vi "TemperatureSensorStart.vi"(0 "Device Info":T1={"Serial Number"=-1, "Channel"=0, "Port"=0}, 1 "Data Interval":i32=-1, 2 "Change Trigger":dbl, 5 "ThermocoupleType":u32(ring)=2 items=["THERMOCOUPLE_TYPE_J"=1, "THERMOCOUPLE_TYPE_K"=2, "THERMOCOUPLE_TYPE_E"=3, "THERMOCOUPLE_TYPE_T"=4], 7 "RTD Type":u32(ring)=2 items=["RTD_TYPE_PT100_3850"=1, "RTD_TYPE_PT1000_3850"=2, "RTD_TYPE_PT100_3920"=3, "RTD_TYPE_PT1000_3920"=4], 9 "RTD Wire Setup":u32(ring)=3 items=["RTD_WIRE_SETUP_2WIRE"=1, "RTD_WIRE_SETUP_3WIRE"=2, "RTD_WIRE_SETUP_4WIRE"=3], 11 "error in (no error)":errorcluster, 12 "Connection":u16(ring) items=["No Preference", "Remote", "Local"], 13 "Timeout (mSec)":i32=5000) -> (4 "Phidget ID":u64, 6 "Serial Number Return":i32, 10 "Attached?":bool, 15 "error out":errorcluster)   [LabVIEW 2012, in "Phidget Temperature Sensor.lvlib"]
doc: "${TemperatureSensor:StartHeader}"
uses:
  <instrlib>/Phidgets/Phidget Temperature Sensor/Phidget Temperature Sensor.lvlib
  <instrlib>/Phidgets/Phidget Common/Phidget Common.lvlib
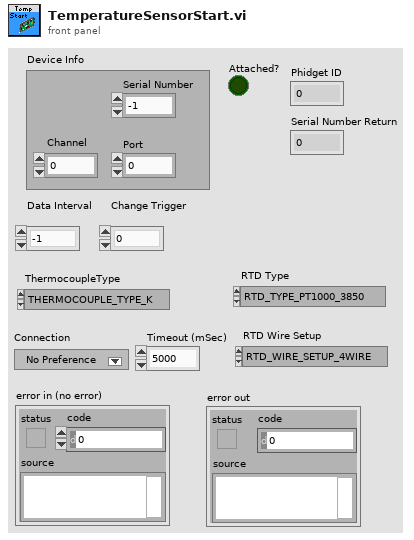
[diagram p1: front panel]
types:
  T1 = cluster{"Serial Number":i32, "Channel":i32, "Port":i32}
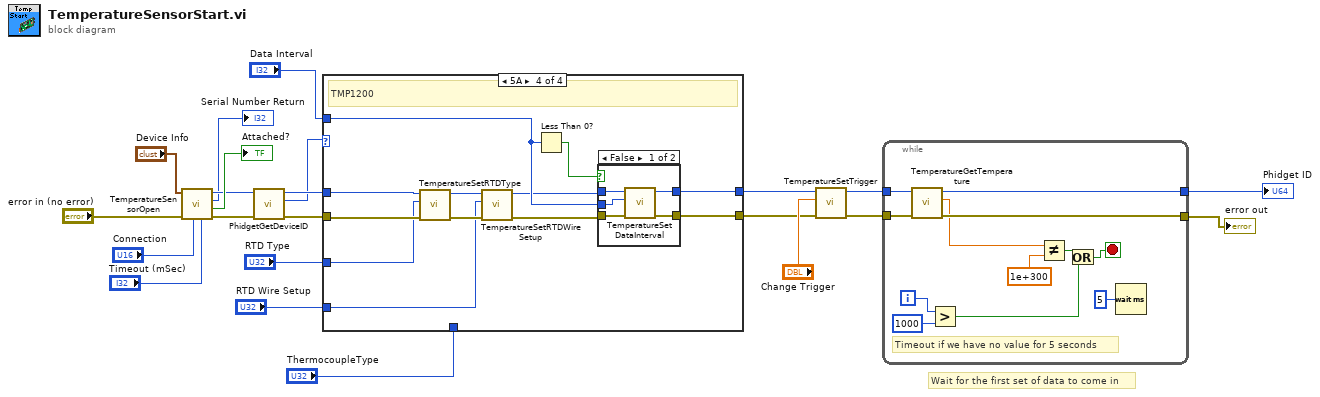
[diagram p0: block diagram]
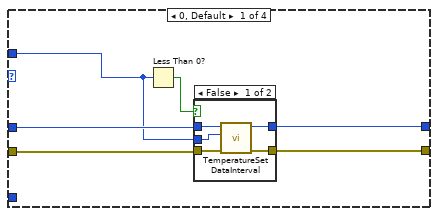
[diagram p2: hidden frame]
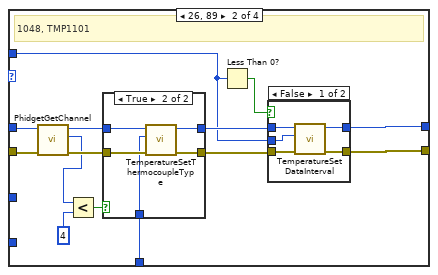
[diagram p4: hidden frame]
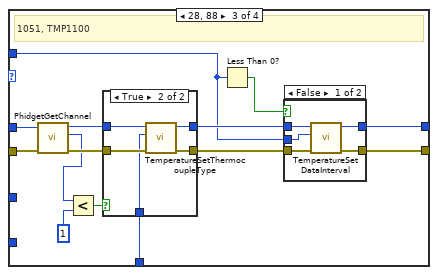
[diagram p7: hidden frame]
diagram:
  # "Wait for the first set of data to come in"
  n1 = call <instrlib>:"TemperatureSensorOpen.vi"("Timeout (mSec)"="Timeout (mSec)", "Connection"="Connection", "error in"="error in (no error)", "Device Info"="Device Info") -> ("error out"=w19:errorcluster, "Attached?"=→"Attached?":bool, "Serial Number Return"=→"Serial Number Return":i32, "Phidget ID"=w18:u64)  [unwired: 4 in]
  n2 = call <instrlib>:"PhidgetGetDeviceID.vi"("error in (no error)"=w19, "Device In"=w18) -> ("error out"=w12:errorcluster, "Devie IDs"=w11:u32, "Device Out"=w13:u64)  [unwired: 6 in]
  n3 = case shown="5A" w11 {
    tunnel: w13 -> [w27 w49 w72 w99]
    tunnel: w12 -> [w26 w48 w71 w96]
    tunnel: [w24 w36 w64 w100] -> w4
    tunnel: [w25 w37 w65 w101] -> w5
    tunnel: "ThermocoupleType" -> [_ w42 w70 _]
    tunnel: "Data Interval" -> [w23 w38 w67 w102]
    tunnel: "RTD Type" -> [_ _ _ w93]
    tunnel: "RTD Wire Setup" -> [_ _ _ w92]
    frame 0, Default {
      n4 = Less Than 0?(x=w23) -> (x < 0?=w28:bool)
      n5 = case shown="False" w28 {
        tunnel: w27 -> [w31 w35]
        tunnel: w26 -> [w33 w34]
        tunnel: [w30 w35] -> w24
        tunnel: [w29 w34] -> w25
        tunnel: w23 -> [w32 _]
        frame False {
          n6 = call <instrlib>:"TemperatureSetDataInterval.vi"("error in (no error)"=w33, "Interval"=w32, "Device In"=w31) -> ("error out"=w29:errorcluster, "Device Out"=w30:u64)  [unwired: 6 in]
        }
        frame True {
        }
      }
    }
    frame 26, 89 {
      # "1048, TMP1101"
      n7 = call <instrlib>:"PhidgetGetChannel.vi"("error in (no error)"=w48, "Device In"=w49) -> ("error out"=w47:errorcluster, "Channel"=w46:i32, "Device Out"=w43:u64)  [unwired: 6 in]
      n8 = Less?(x=w46, y=4 ("index")) -> (x < y?=w44:bool)
      n9 = case shown="True" w44 {
        tunnel: w47 -> [w58 w63]
        tunnel: [w58 w62] -> w40
        tunnel: [w57 w61] -> w39
        tunnel: w43 -> [w57 w60]
        tunnel: w42 -> [_ w59]
        frame False {
        }
        frame True {
          n10 = call <instrlib>:"TemperatureSetThermocoupleType.vi"("error in (no error)"=w63, "ThermocoupleType"=w59, "Device In"=w60) -> ("error out"=w62:errorcluster, "Device Out"=w61:u64)  [unwired: 6 in]
        }
      }
      n11 = Less Than 0?(x=w38) -> (x < 0?=w41:bool)
      n12 = case shown="False" w41 {
        tunnel: w39 -> [w52 w56]
        tunnel: w40 -> [w54 w55]
        tunnel: [w51 w56] -> w36
        tunnel: [w50 w55] -> w37
        tunnel: w38 -> [w53 _]
        frame False {
          n13 = call <instrlib>:"TemperatureSetDataInterval.vi"("error in (no error)"=w54, "Interval"=w53, "Device In"=w52) -> ("error out"=w50:errorcluster, "Device Out"=w51:u64)  [unwired: 6 in]
        }
        frame True {
        }
      }
    }
    frame 28, 88 {
      # "1051, TMP1100"
      n14 = call <instrlib>:"PhidgetGetChannel.vi"("error in (no error)"=w71, "Device In"=w72) -> ("error out"=w77:errorcluster, "Channel"=w76:i32, "Device Out"=w73:u64)  [unwired: 6 in]
      n15 = Less?(x=w76, y=1 ("index")) -> (x < y?=w74:bool)
      n16 = case shown="True" w74 {
        tunnel: w77 -> [w86 w91]
        tunnel: [w86 w90] -> w66
        tunnel: [w85 w89] -> w68
        tunnel: w73 -> [w85 w88]
        tunnel: w70 -> [_ w87]
        frame False {
        }
        frame True {
          n17 = call <instrlib>:"TemperatureSetThermocoupleType.vi"("error in (no error)"=w91, "ThermocoupleType"=w87, "Device In"=w88) -> ("error out"=w90:errorcluster, "Device Out"=w89:u64)  [unwired: 6 in]
        }
      }
      n18 = Less Than 0?(x=w67) -> (x < 0?=w69:bool)
      n19 = case shown="False" w69 {
        tunnel: w68 -> [w80 w84]
        tunnel: w66 -> [w82 w83]
        tunnel: [w79 w84] -> w64
        tunnel: [w78 w83] -> w65
        tunnel: w67 -> [w81 _]
        frame False {
          n20 = call <instrlib>:"TemperatureSetDataInterval.vi"("error in (no error)"=w82, "Interval"=w81, "Device In"=w80) -> ("error out"=w78:errorcluster, "Device Out"=w79:u64)  [unwired: 6 in]
        }
        frame True {
        }
      }
    }
    frame 90 {
      # "TMP1200"
      n21 = call <instrlib>:"TemperatureSetRTDType.vi"("error in (no error)"=w96, "RTD Type"=w93, "Device In"=w99) -> ("error out"=w97:errorcluster, "Device Out"=w98:u64)  [unwired: 6 in]
      n22 = call <instrlib>:"TemperatureSetRTDWireSetup.vi"("error in (no error)"=w97, "RTD Wire Setup"=w92, "Device In"=w98) -> ("error out"=w94:errorcluster, "Device Out"=w95:u64)  [unwired: 6 in]
      n23 = Less Than 0?(x=w102) -> (x < 0?=w103:bool)
      n24 = case shown="False" w103 {
        tunnel: w95 -> [w106 w110]
        tunnel: w94 -> [w108 w109]
        tunnel: [w105 w110] -> w100
        tunnel: [w104 w109] -> w101
        tunnel: w102 -> [w107 _]
        frame False {
          n25 = call <instrlib>:"TemperatureSetDataInterval.vi"("error in (no error)"=w108, "Interval"=w107, "Device In"=w106) -> ("error out"=w104:errorcluster, "Device Out"=w105:u64)  [unwired: 6 in]
        }
        frame True {
        }
      }
    }
  }
  n26 = call <instrlib>:"TemperatureSetTrigger.vi"("error in (no error)"=w5, "Trigger"="Change Trigger", "Device In"=w4) -> ("error out"=w14:errorcluster, "Device Out"=w15:u64)  [unwired: 6 in]
  n27 = while {
    tunnel: w15 -> [w120]
    tunnel: w14 -> [w119]
    tunnel: [w117] -> w17
    tunnel: [w118] -> w21
    i -> [w112]
    stop <- w114 stop-if-true
    # "Timeout if we have no value for 5 seconds"
    n28 = call <instrlib>:"TemperatureGetTemperature.vi"("error in (no error)"=w119, "Device In"=w120) -> ("error out"=w118:errorcluster, "temperature"=w111:dbl, "Device Out"=w117:u64)  [unwired: 6 in]
    n29 = Greater?(x=w112, y=1000) -> (0:w115:bool)
    n30 = Not Equal?(x=w111, y=1e+300) -> (x != y?=w116:bool)
    n31 = Or(x=w116, y=w115) -> (x .or. y?=w114:bool)
    n32 = Wait (ms)(milliseconds to wait=u32 5) -> ()  [unwired: 1 out]
  }
  "error out" <- w21
  "Phidget ID" <- w17
